vi "ElevatorPID.vi"(9 "Elevator Setpoint":dbl format="%.2f") -> (15 "At Setpoint":bool)   [LabVIEW 2014]
uses:
  Robot Global Data.vi
  <vilib>/addons/control/pid/pid.llb/PID (DBL).vi
  <vilib>/addons/control/pid/NI_PID_pid.lvlib
  <vilib>/addons/control/pid/NI_PID_autopid.lvlib
panel:
  out "tuning completed?":bool
  out "Encoder Graph":dbl[](graph)
  in  "Elevator Setpoint":dbl format="%.2f"
  out "Encoder Graph":dbl[](graph)
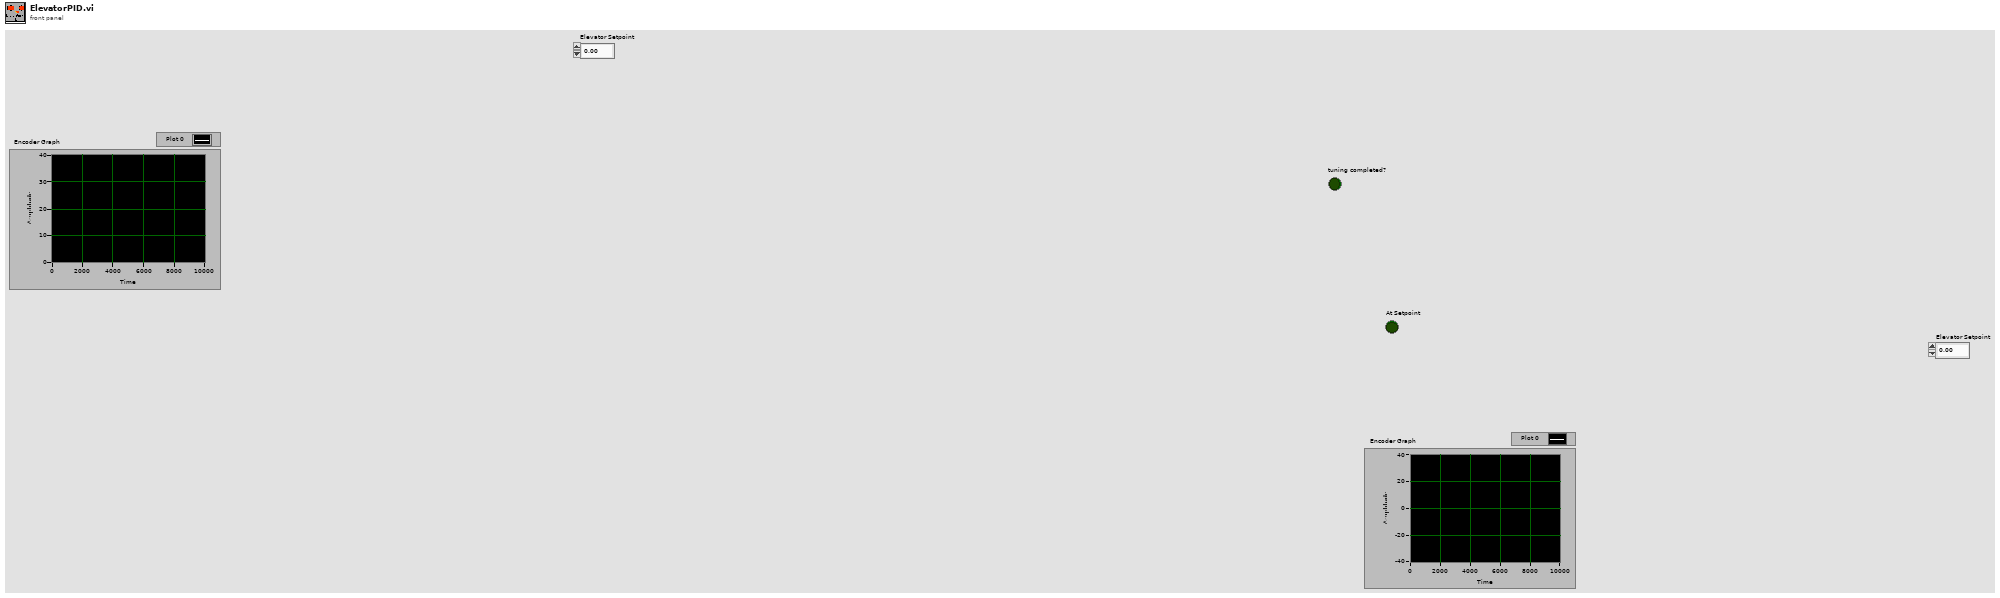
[diagram p1: front panel]
types:
  T1 = cluster{"controller type":u16, "relay cycles":i32, "relay amplitude":dbl, "control specification":u16, "PV noise level":dbl}
  T2 = cluster{"proportional gain (Kc)":dbl, "integral time (Ti, min)":dbl, "derivative time (Td, min)":dbl}
  T3 = typedef "WPI_EncoderDevRef.ctl" = cluster{"DevStatus":errorcluster, "EncoderIndex":T4, "CounterIndex":T5, "DistancePerCount":dbl, "Decoding Type":T6}
  T4 = typedef "FPGA_EncoderIdx.ctl" = enum8{"Enc 0", "Enc 1", "Enc 2", "Enc 3", "Enc 4", "Enc 5", "Enc 6", "Enc 7", "Invalid"}
  T5 = typedef "FPGA_CounterCtrSystemIndex.ctl" = enum8{"Ctr 0", "Ctr 1", "Ctr 2", "Ctr 3", "Ctr 4", "Ctr 5", "Ctr 6", "Ctr 7", "Invalid"}
  T6 = typedef "WPI_EncoderType.ctl" = enum16{"1x", "2x", "4x"}
  T7 = typedef "WPI_MotorControlDeviceRef.ctl" = cluster{"DeviceStatus":errorcluster, "Type":T8, "PWM":cluster{"Controller":T9, "PWM Channel":T10, "DeadBand":T11}, "CAN":cluster{"Device Number":u8, "Control Mode":T12, "Semaphore":T13, "Max Vout":dbl, "TalonSRX Control Mode":T14}, "Invert":bool, "TransformRef":T15, "InvTransformRef":T15}
  T8 = typedef "WPI_MotorControlType.ctl" = enum16{"PWM", "CAN", "CANTalonSRX"}
  T9 = typedef "FPGA_TypedefDigitalModule.ctl" = enum16{"Controller 1"}
  T10 = typedef "FPGA_DIOPWMChannel.ctl" = enum8{"PWM 0", "PWM 1", "PWM 2", "PWM 3", "PWM 4", "PWM 5", "PWM 6", "PWM 7", "PWM 8", "PWM 9", "PWM MXP 0", "PWM MXP 1", "PWM MXP 2", "PWM MXP 3", "PWM MXP 4", "PWM MXP 5", "PWM MXP 6", "PWM MXP 7", "PWM MXP 8", "PWM MXP 9", "Invalid"}
  T11 = typedef "WPI_PWMDeadband.ctl" = cluster{"Name":string, "maxPositivePwm":i32, "minPositivePwm":i32, "centerPwm":i32, "maxNegativePwm":i32, "minNegativePwm":i32, "angularRange":u16}
  T12 = typedef "WPI_CANJaguar_ControlMode.ctl" = enum8{"Percent VBus", "Current", "Speed", "Position", "Voltage"}
  T13 = typedef "Semaphore RefNum" = refnum<k1>
  T14 = typedef "WPI_CANTalonSRX_APIControlMode.ctl" = enum8{"Percent VBus", "Speed", "Position", "Slave", "Unchanged / Invalid"}
  T15 = typedef "WPI_PWMTransform_ConPane.ctl" = refnum<vi>
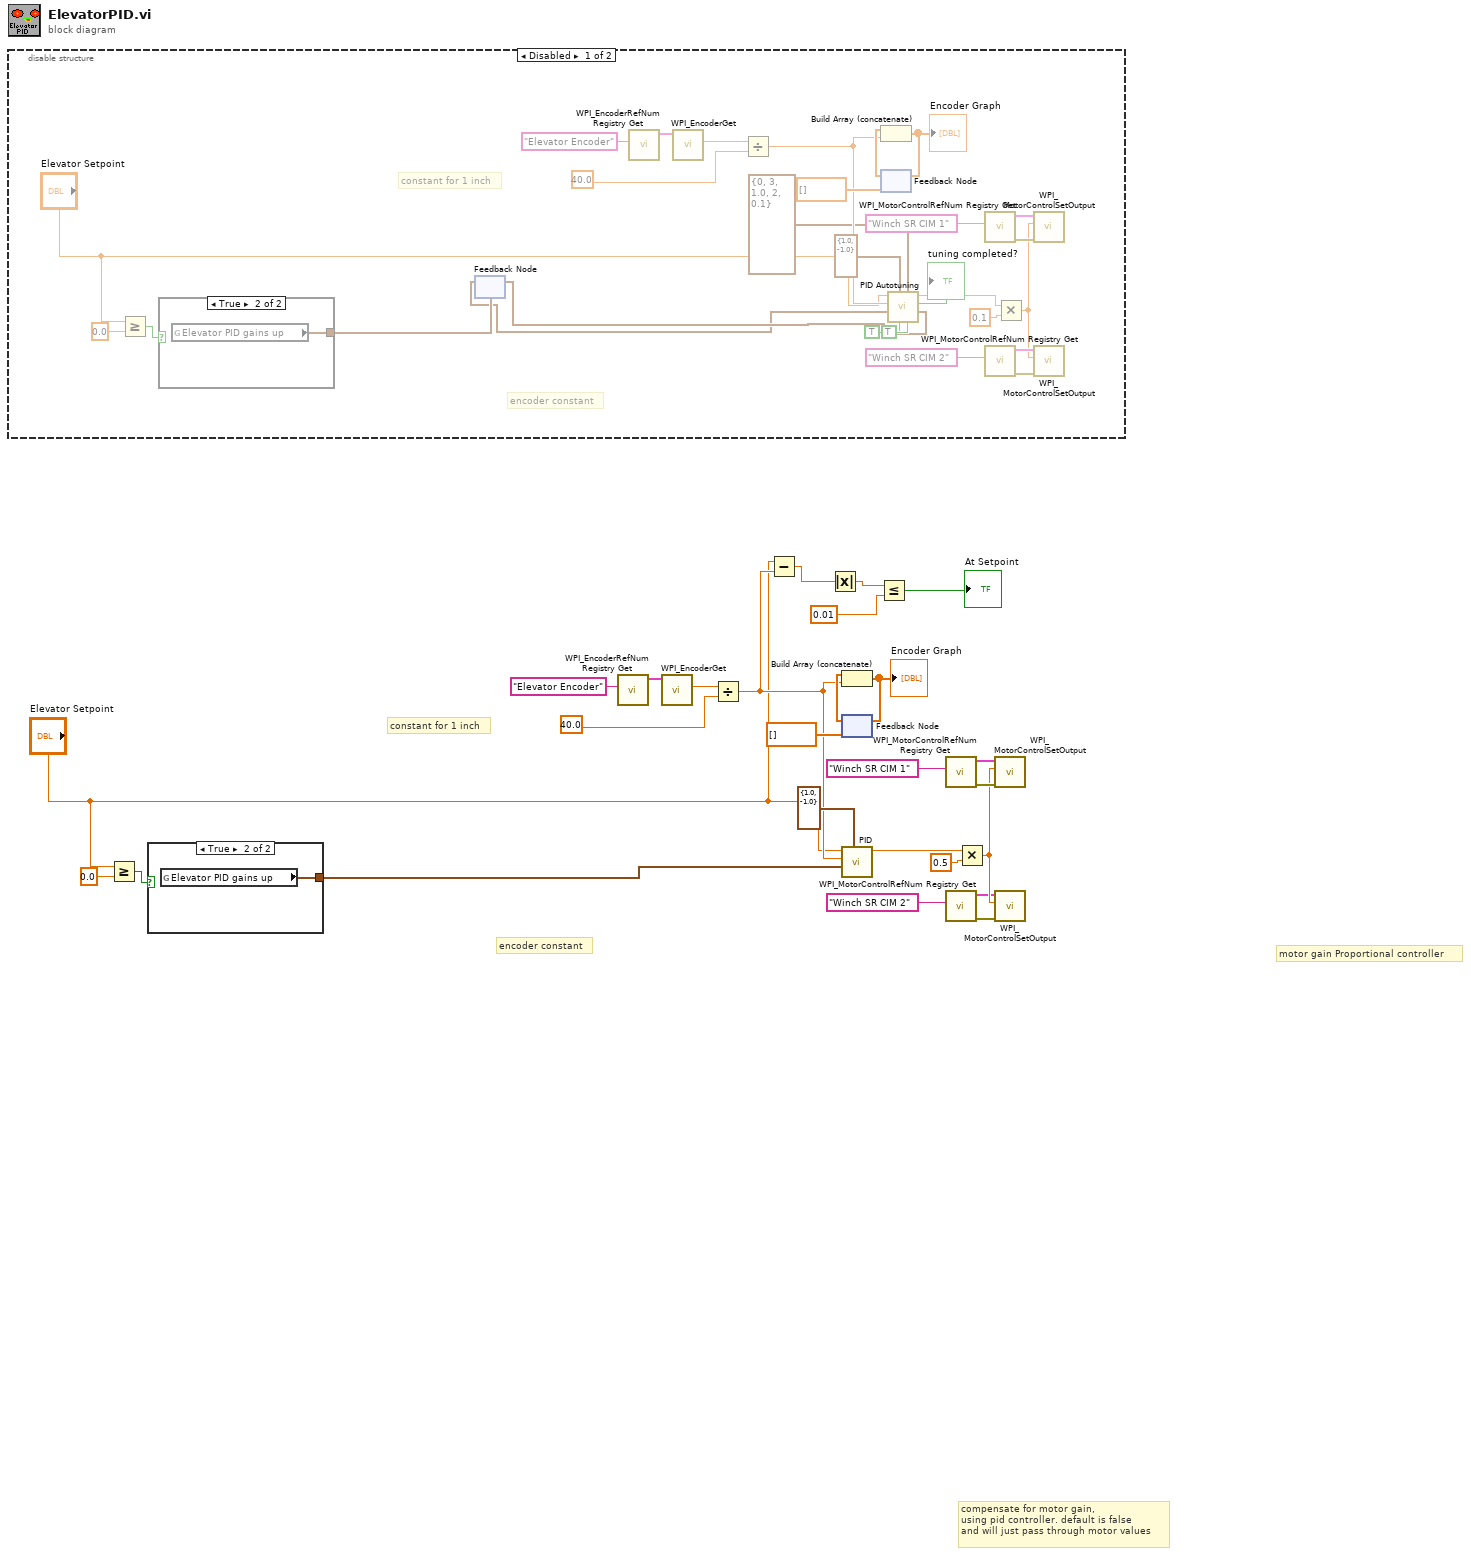
[diagram p0: block diagram]
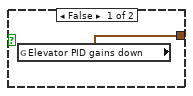
[diagram p2: hidden frame]
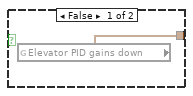
[diagram p3: hidden frame]
diagram:
  # "constant for 1 inch"
  # "encoder constant"
  # "motor gain Proportional controller"
  # "compensate for motor gain,\nusing pid controller. default is false\nand will just pass through motor values"
  n1 = disable-structure shown="Disabled" {
    frame Disabled {
      # "constant for 1 inch"
      # "encoder constant"
      n2 = Greater Or Equal?(x="Elevator Setpoint", y=0.0) -> (x >= y?=w38:bool)
      n3 = case shown="True" w38 {
        tunnel: [w55 w56] -> w31
        frame False {
          n4 = global read "Robot Global Data.vi" "Elevator PID gains down"() -> (w55:T2)
        }
        frame True {
          n5 = global read "Robot Global Data.vi" "Elevator PID gains up"() -> (w56:T2)
        }
      }
      n6 = feedback #1(w31) -> (w29:T2)
      n7 = call <vilib>:"WPI_EncoderRefNum Registry Get.vi"("refnum name"="Elevator Encoder") -> ("EncoderDevRef"=w53:T3)  [unwired: 9 in, 1 out]
      n8 = call <vilib>:"WPI_EncoderGet.vi"("EncoderDevRef"=w53) -> ("Distance"=w52:dbl)  [unwired: 5 in, 5 out]
      n9 = Divide(x=w52, y=40.0) -> (x/y=w37:dbl)
      n10 = feedback #2(dbl[] []) -> (w49:dbl[])
      n11 = Build Array (concatenate)(w49, w37) -> (w50:dbl[])
      "Encoder Graph" <- w50
      n12 = feedback-in #2(w50) -> ()
      n13 = call <vilib>:"PID Autotuning.vi"("autotune? (F)"=TRUE, "autotuning parameters"=T1 {"controller type"=0, "relay cycles"=3, "relay amplitude"=1.0, "control specification"=2, "PV noise level"=0.1}, "reinitialize? (F)"=TRUE, "output range"=cluster{"output high":dbl, "output low":dbl} {"output high"=1.0, "output low"=-1.0}, "PID gains"=w29, "process variable"=w37, "setpoint"="Elevator Setpoint") -> ("PID gains out"=w30:T2, "tuning completed?"=→"tuning completed?":bool, "output"=w35:dbl)  [unwired: 1 in, 1 out]
      n14 = feedback-in #1(w30) -> ()
      n15 = call <vilib>:"WPI_MotorControlRefNum Registry Get.vi"("refnum name"="Winch SR CIM 1") -> ("error out"=w46:errorcluster, "MotorControlDevRef"=w45:T7)  [unwired: 9 in]
      n16 = call <vilib>:"WPI_MotorControlRefNum Registry Get.vi"("refnum name"="Winch SR CIM 2") -> ("error out"=w43:errorcluster, "MotorControlDevRef"=w42:T7)  [unwired: 9 in]
      n17 = Multiply(x=w35, y=0.1) -> (x*y=w41:dbl)
      n18 = call <vilib>:"WPI_MotorControlSetOutput.vi"("error in (no error)"=w46, "Output"=w41, "MotorControlDevRef"=w45) -> ()  [unwired: 6 in, 3 out]
      n19 = call <vilib>:"WPI_MotorControlSetOutput.vi"("error in (no error)"=w43, "Output"=w41, "MotorControlDevRef"=w42) -> ()  [unwired: 6 in, 3 out]
    }
    frame Enabled {
    }
  }
  n20 = Greater Or Equal?(x="Elevator Setpoint", y=0.0) -> (x >= y?=w11:bool)
  n21 = case shown="True" w11 {
    tunnel: [w57 w58] -> w22
    frame False {
      n22 = global read "Robot Global Data.vi" "Elevator PID gains down"() -> (w57:T2)
    }
    frame True {
      n23 = global read "Robot Global Data.vi" "Elevator PID gains up"() -> (w58:T2)
    }
  }
  n24 = call <vilib>:"WPI_EncoderRefNum Registry Get.vi"("refnum name"="Elevator Encoder") -> ("EncoderDevRef"=w25:T3)  [unwired: 9 in, 1 out]
  n25 = call <vilib>:"WPI_EncoderGet.vi"("EncoderDevRef"=w25) -> ("Distance"=w24:dbl)  [unwired: 5 in, 5 out]
  n26 = Divide(x=w24, y=40.0) -> (x/y=w9:dbl)
  n27 = Subtract(x="Elevator Setpoint", y=w9) -> (x-y=w7:dbl)
  n28 = Absolute Value(x=w7) -> (abs(x)=w6:dbl)
  n29 = feedback #3(dbl[] []) -> (w20:dbl[])
  n30 = Build Array (concatenate)(w20, w9) -> (w21:dbl[])
  "Encoder Graph" <- w21
  n31 = feedback-in #3(w21) -> ()
  n32 = call-poly <vilib>:"PID.vi"("output range"=cluster{"output high":dbl, "output low":dbl} {"output high"=1.0, "output low"=-1.0}, "PID gains"=w22, "process variable"=w9, "setpoint"="Elevator Setpoint") -> ("output"=w13:dbl)  [unwired: 6 in, 1 out]
  n33 = Less Or Equal?(x=w6, y=0.01) -> (x <= y?=→"At Setpoint":bool)
  n34 = call <vilib>:"WPI_MotorControlRefNum Registry Get.vi"("refnum name"="Winch SR CIM 1") -> ("error out"=w17:errorcluster, "MotorControlDevRef"=w16:T7)  [unwired: 9 in]
  n35 = call <vilib>:"WPI_MotorControlRefNum Registry Get.vi"("refnum name"="Winch SR CIM 2") -> ("error out"=w2:errorcluster, "MotorControlDevRef"=w1:T7)  [unwired: 9 in]
  n36 = Multiply(x=w13, y=0.5) -> (x*y=w15:dbl)
  n37 = call <vilib>:"WPI_MotorControlSetOutput.vi"("error in (no error)"=w17, "Output"=w15, "MotorControlDevRef"=w16) -> ()  [unwired: 6 in, 3 out]
  n38 = call <vilib>:"WPI_MotorControlSetOutput.vi"("error in (no error)"=w2, "Output"=w15, "MotorControlDevRef"=w1) -> ()  [unwired: 6 in, 3 out]
